vi "factoriel2(while).vi"() -> ()   [LabVIEW 2014]
panel:
  out "nbr iteration":dbl
  out "resultat":dbl
  in  "factoriel":dbl
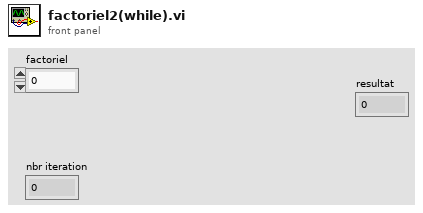
[diagram p1: front panel]
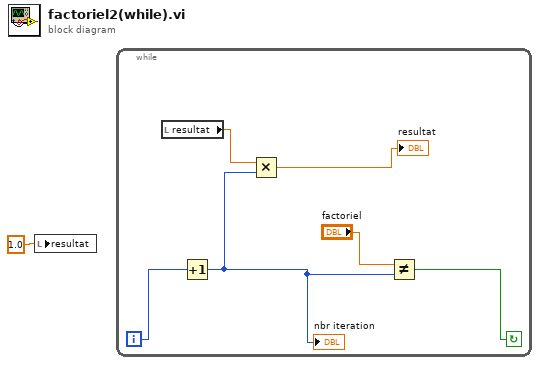
[diagram p0: block diagram]
diagram:
  n1 = local write "resultat"(1.0) -> ()
  n2 = while {
    i -> [w7]
    stop <- w2 continue-if-true
    n3 = local read "resultat"() -> (w6:dbl)
    n4 = Increment(x=w7) -> (x+1=w3:i32)
    "nbr iteration" <- w3
    n5 = Multiply(x=w6, y=w3) -> (x*y=→"resultat":dbl)
    n6 = Not Equal?(x="factoriel", y=w3) -> (x != y?=w2:bool)
  }
